vi "ActionVIOnCompile.vi"(8 "error in (no error)":errorcluster, 11 "Device Item Ref in":T1 format="%.0x") -> (0 "error out":errorcluster)   [LabVIEW 2019, in "Profile Interpolation System Explorer.lvlib"]
uses:
  Profile Interpolation System Explorer.lvlib
  <vilib>/NI VeriStand/Custom Device API/Custom Device Item Ref.ctl
  Shared/Types/Compiled.Settings.ctl
  <vilib>/NI VeriStand/Custom Device API/Custom Device Target Type.ctl
  Shared/Types/FG Action.ctl
  Shared/SubVIs/Constants.vi
  <vilib>/NI VeriStand/Custom Device API/NI VeriStand - Get Item Property.vi
  <vilib>/NI VeriStand/Custom Device API/Get Item Property (Path).vi
  <vilib>/NI VeriStand/Custom Device API/Get Item Property (Boolean).vi
  <vilib>/NI VeriStand/Custom Device API/Set Item Property (Path).vi
  <vilib>/NI VeriStand/Custom Device API/Set Item Property (Boolean).vi
  <vilib>/NI VeriStand/Custom Device Tools/Custom Device Utility Library/NI VeriStand - Search for Item by Name.vi
  <vilib>/NI VeriStand/Custom Device API/Set Item Property (Variant).vi
  <vilib>/NI VeriStand/Custom Device Tools/Custom Device Utility Library/Custom Device Utility Library.lvlib
  <vilib>/NI VeriStand/Custom Device API/Custom Device API.lvlib
  <vilib>/NI/NIVS Inline Async API/_Data Access System Explorer/Data Access System Explorer.lvlib
  Shared/Profile Interpolation Shared.lvlib
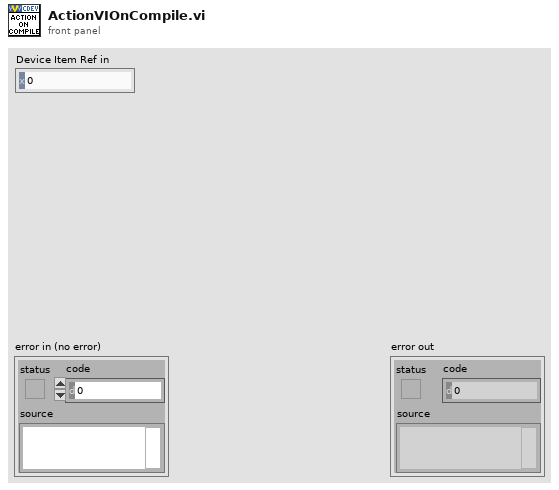
[diagram p1: front panel]
types:
  T1 = typedef "Custom Device API.lvlib/Custom Device Item Ref.ctl" = u64
  T2 = typedef "Profile Interpolation Shared.lvlib/FG Action.ctl" = enum8{"GET", "SET"}
  T3 = enum16{"Output/Write", "Input/Read", "Input/ReadWrite"}
  T4 = cluster{"Name":string, "Type":enum16{"Output/Write", "Input/Read", "Input/ReadWrite"}, "VS Refs":T1[]}
  T5 = typedef "Profile Interpolation Shared.lvlib/Compiled.Settings.ctl" = cluster{"Name":string, "Create Limit Channels?":bool, "Profiles []":cluster{"Profile":dbl[][]}[], "Target.Type":T6}
  T6 = typedef "Custom Device API.lvlib/Custom Device Target Type.ctl" = enum16{"PharLap", "VxWorks", "Windows", "Linux_32_ARM", "Linux_x64"}
  T7 = typedef "Profile Interpolation Shared.lvlib/Interpolation Settings.ctl" = cluster{"Interpolation File":path, "Create Limit Channels?":bool}
  T8 = typedef "Custom Device API.lvlib/Custom Device Item Info.ctl" = cluster{"Name":string, "Is Channel":bool, "GUID":string, "Is Waveform":bool}
  T9 = cluster{"Name":string, "Type":enum16{"Output/Write", "Input/Read", "Input/ReadWrite"}, "VS Refs":T1[]}[]
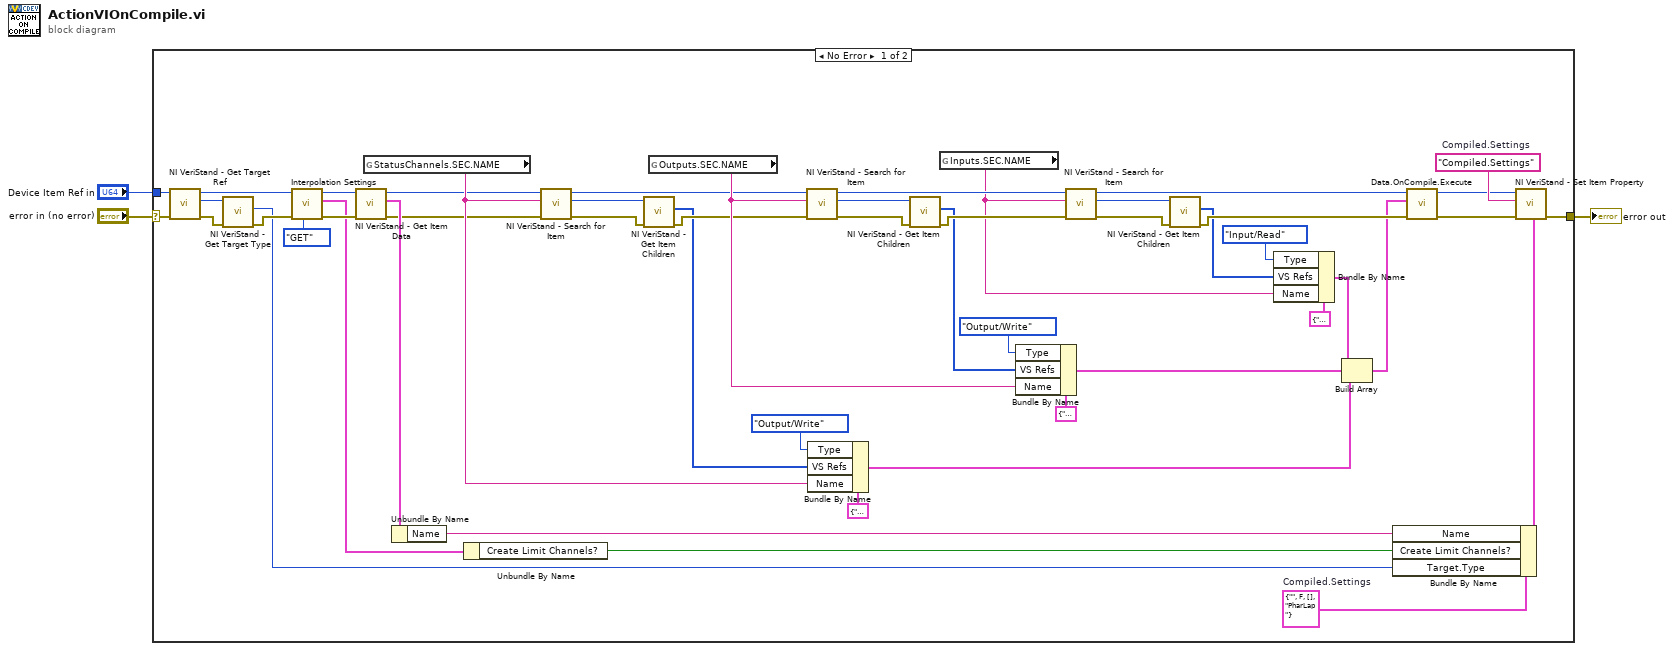
[diagram p0: block diagram]
diagram:
  n1 = case shown="No Error" "error in (no error)" {
    selector: "error in (no error)" -> [w9 w54]
    tunnel: [w47 w54] -> w2
    tunnel: "Device Item Ref in" -> [w7 _]
    frame No Error {
      w32 = T5 {"Name"="", "Create Limit Channels?"=FALSE, "Profiles []"=[], "Target.Type"=enum."PharLap"}  # Compiled.Settings
      w49 = "Compiled.Settings"  # Compiled.Settings
      n2 = call <vilib>:"NI VeriStand - Get Target Ref.vi"("error in"=w9, "Item Ref in"=w7) -> ("error out"=w10:errorcluster, "Target Ref"=w6:T1, "Item Ref out"=w5:T1)  [unwired: 6 in, 1 out]
      n3 = call <vilib>:"NI VeriStand - Get Target Type.vi"("error in (no error)"=w10, "Item Ref in"=w6) -> ("error out"=w8:errorcluster, "Target Type"=w4:T6)  [unwired: 7 in, 1 out]
      n4 = call "Interpolation Settings.vi"("Action"=FG_Action."GET", "error in (no error)"=w8, "Item Ref"=w5) -> ("error out"=w15:errorcluster, "Interpolation Settings out"=w12:T7, "Item Ref out"=w14:T1)  [unwired: 6 in]
      n5 = call <vilib>:"NI VeriStand - Get Item Data.vi"("error in (no error)"=w15, "Item Ref in"=w14) -> ("error out"=w22:errorcluster, "Item Info"=w46:T8, "Item Ref out"=w23:T1)  [unwired: 6 in, 1 out]
      n6 = global read "Constants.vi" "StatusChannels.SEC.NAME"() -> (w25:string)
      n7 = Unbundle By Name(w46) -> ("Name"=w45:string)
      n8 = Unbundle By Name(w12) -> ("Create Limit Channels?"=w11:bool)
      n9 = call-poly <vilib>:"NI VeriStand - Search for Item.vi"("error in"=w22, "Item Name"=w25, "Section Ref in"=w23) -> ("error out"=w29:errorcluster, "Item Ref"=w28:T1, "Section Ref out"=w24:T1)  [unwired: 5 in, 1 out]
      n10 = call <vilib>:"NI VeriStand - Get Item Children.vi"("error in (no error)"=w29, "Item Ref in"=w28) -> ("error out"=w21:errorcluster, "Child Refs"=w20:T1[])  [unwired: 6 in, 2 out]
      n11 = global read "Constants.vi" "Outputs.SEC.NAME"() -> (w34:string)
      n12 = call-poly <vilib>:"NI VeriStand - Search for Item.vi"("error in"=w21, "Item Name"=w34, "Section Ref in"=w24) -> ("error out"=w53:errorcluster, "Item Ref"=w52:T1, "Section Ref out"=w38:T1)  [unwired: 5 in, 1 out]
      n13 = Bundle By Name(cluster=T4 {"Name"="", "Type"=enum."Output/Write", "VS Refs"=[]} ("Group"), "Type"=T3."Output/Write", "VS Refs"=w20, "Name"=w25) -> (w17:T4)
      n14 = call <vilib>:"NI VeriStand - Get Item Children.vi"("error in (no error)"=w53, "Item Ref in"=w52) -> ("error out"=w37:errorcluster, "Child Refs"=w31:T1[])  [unwired: 6 in, 2 out]
      n15 = global read "Constants.vi" "Inputs.SEC.NAME"() -> (w33:string)
      n16 = Bundle By Name(cluster=T4 {"Name"="", "Type"=enum."Output/Write", "VS Refs"=[]} ("Group"), "Type"=T3."Output/Write", "VS Refs"=w31, "Name"=w34) -> (w18:T4)
      n17 = call-poly <vilib>:"NI VeriStand - Search for Item.vi"("error in"=w37, "Item Name"=w33, "Section Ref in"=w38) -> ("error out"=w50:errorcluster, "Item Ref"=w51:T1, "Section Ref out"=w39:T1)  [unwired: 5 in, 1 out]
      n18 = call <vilib>:"NI VeriStand - Get Item Children.vi"("error in (no error)"=w50, "Item Ref in"=w51) -> ("error out"=w40:errorcluster, "Child Refs"=w30:T1[])  [unwired: 6 in, 2 out]
      n19 = Bundle By Name(cluster=T4 {"Name"="", "Type"=enum."Output/Write", "VS Refs"=[]} ("Group"), "Type"=T3."Input/Read", "VS Refs"=w30, "Name"=w33) -> (w19:T4)
      n20 = Build Array(w19, w18, w17) -> (w16:T9)
      n21 = Bundle By Name(cluster=w32, "Name"=w45, "Create Limit Channels?"=w11, "Target.Type"=w4) -> (w48:T5)
      n22 = call <vilib>:"Data.OnCompile.Execute.vi"("error in"=w40, "VS Ref Groups"=w16, "Custom Device Ref"=w39) -> ("error out"=w36:errorcluster, "Custom Device Ref"=w35:T1)  [unwired: 7 in]
      n23 = call-poly <vilib>:"NI VeriStand - Set Item Property.vi"("error in (no error)"=w36, "Value"=w48, "Property Name"=w49, "Item Ref in"=w35) -> ("error out"=w47:errorcluster)  [unwired: 5 in, 2 out]
    }
    frame Error {
    }
  }
  "error out" <- w2
